vi "TrendsD03.vi"() -> ()   [LabVIEW 2019, in "D03.lvlib"]
uses:
  D03.lvlib
panel:
  out "No Change":bool
  out "Sudden Change":bool
  out "Decrease":bool
  out "Increase":bool
  out "Previous  ES":dbl
  out "Present  Speed":dbl
  out "Present Error":dbl format="%#.2g"
  out "Previous Error":dbl
  out "Previous  Speed":dbl
  out "Previous PW":dbl caption="Control Information"
  out "Pulse Trends":waveform(i16)[](graph) caption="Waveform Chart - Dark"
  in  "Close":bool
  out "disc name":string="Disc 03 Trends"
  out "dsgs":string="DSGS"
  out "Speed Trend":waveform(dbl)(graph) caption="Waveform Chart - Dark"
  out "Average Trend":waveform(dbl)[](graph) caption="Waveform Chart - Dark"
  out "Live Trend":waveform(dbl)[](graph) caption="Waveform Chart - Dark"
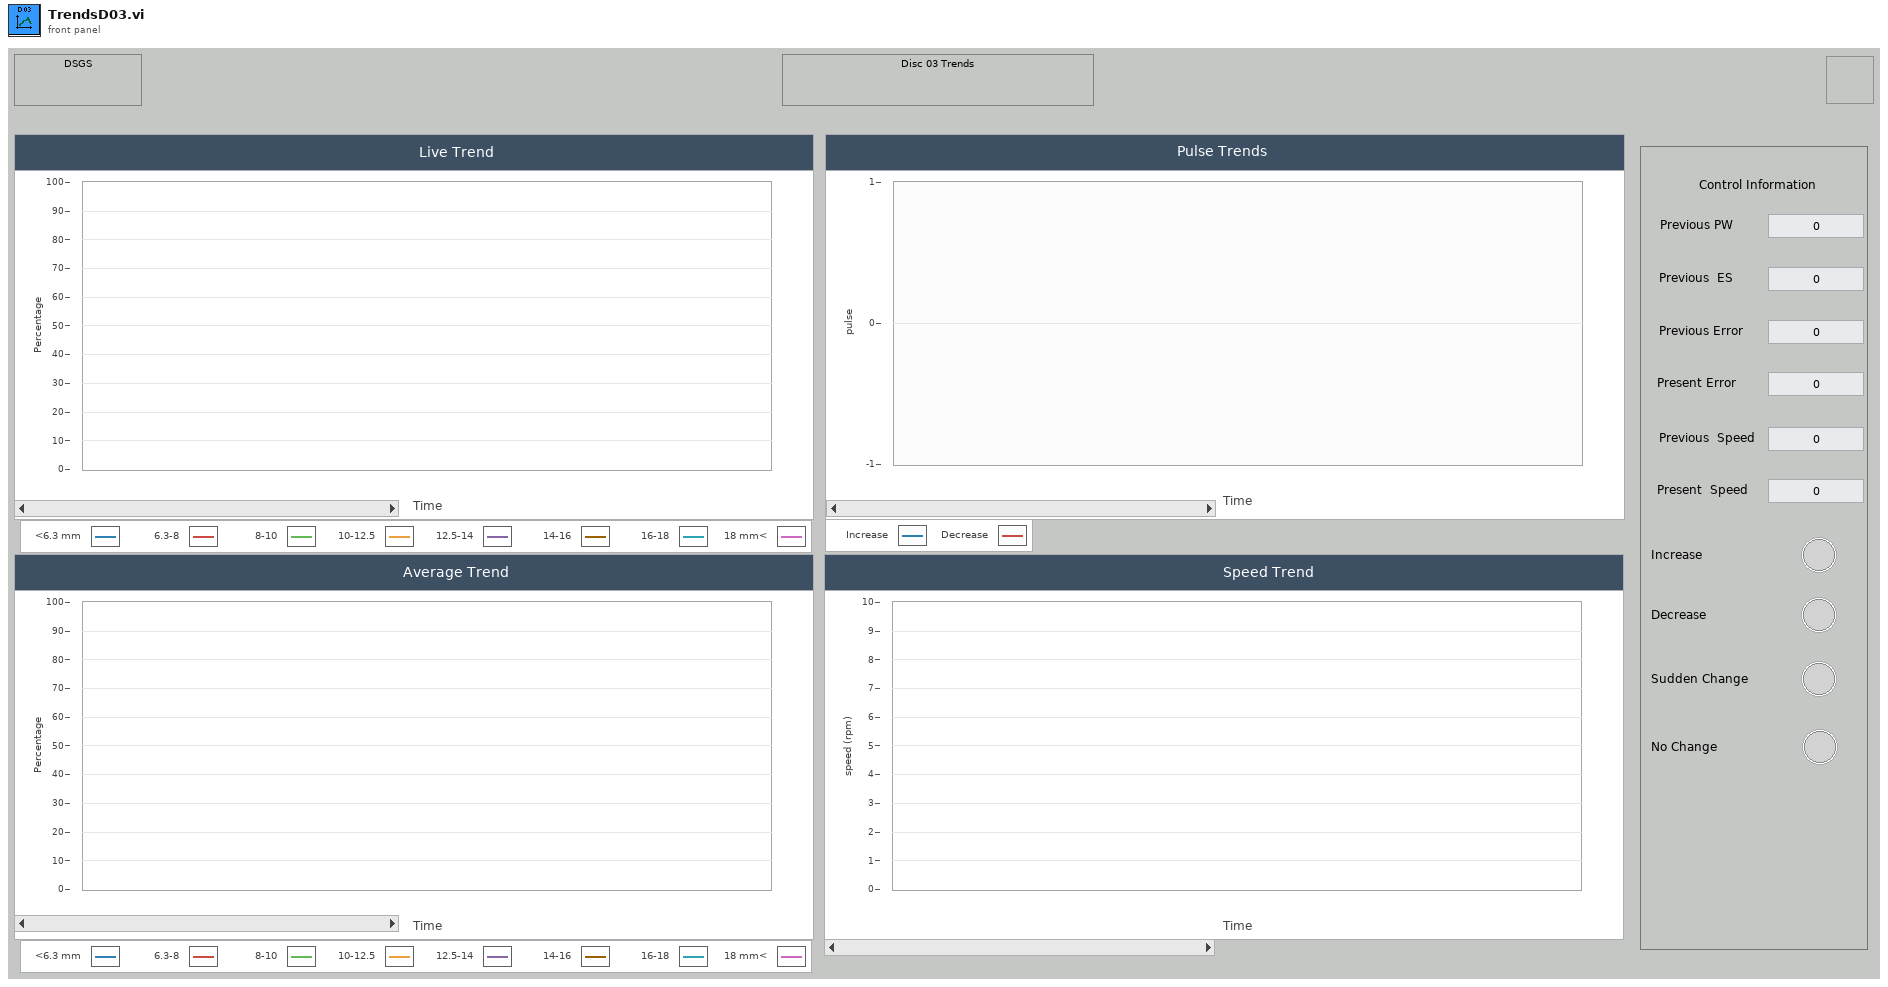
[diagram p1: front panel]
types:
  T1 = cluster{"decrease D28":bool, "increase D28":bool, "no change D28":bool, "sudden change D28":bool, "last error 28":dbl, "previous speed D28":dbl, "pulse width D28":dbl, "slope D28":dbl}
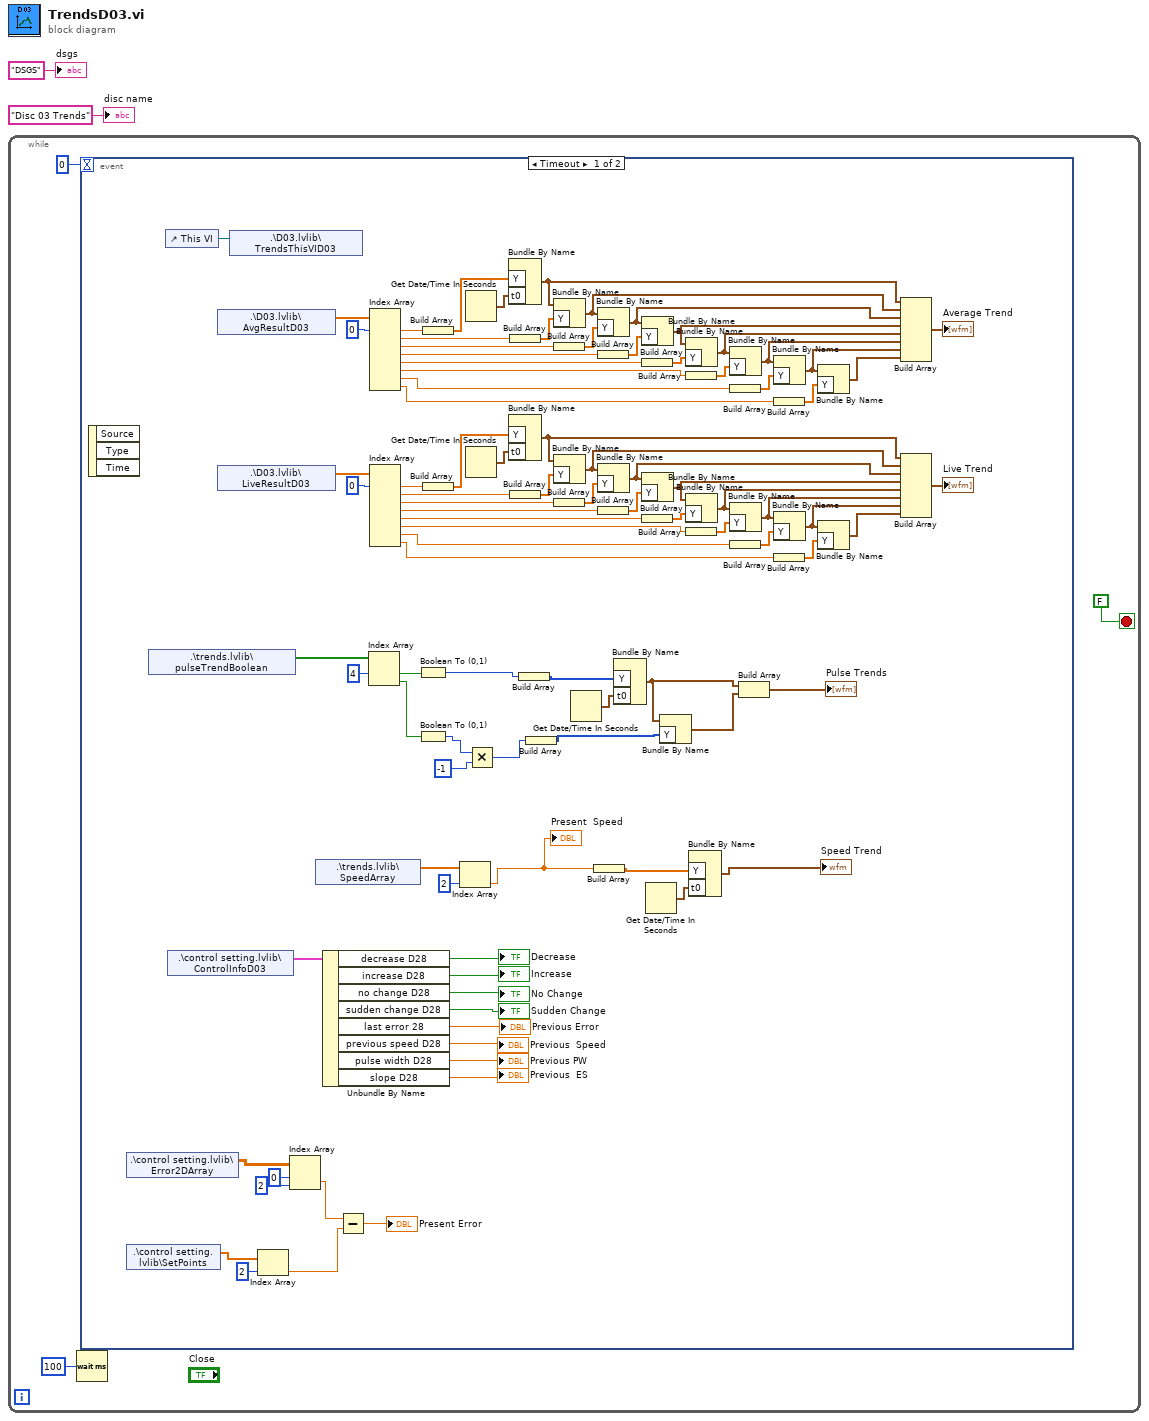
[diagram p0: block diagram]
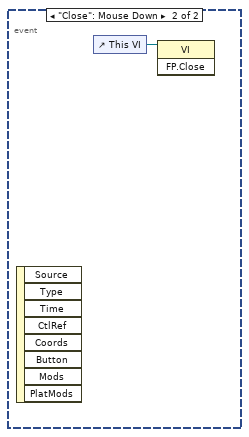
[diagram p2: hidden frame]
diagram:
  n1 = while {
    stop <- FALSE stop-if-true
    n2 = Wait (ms)(milliseconds to wait=u32 100) -> ()  [unwired: 1 out]
    n3 = event shown="[0] Timeout" {
      selector: _ -> [_ _]
      dyn-events: _ -> [_ _]
      timeout: 0 -> [_ _]
      event Timeout {
        n4 = event-data() -> ()  [unwired: 1 in, 3 out]
        n5 = shared-variable ".\\control setting.lvlib\\Error2DArray"() -> (w15:dbl[][])  [unwired: 1 in, 1 out]
        n6 = shared-variable ".\\control setting.lvlib\\SetPoints"() -> (w12:dbl[])  [unwired: 1 in, 1 out]
        n7 = shared-variable ".\\trends.lvlib\\pulseTrendBoolean"() -> (w30:bool[])  [unwired: 1 in, 1 out]
        n8 = control-ref of="This VI"() -> (w43:refnum<vi>)
        n9 = shared-variable ".\\control setting.lvlib\\ControlInfoD03"() -> (w23:T1)  [unwired: 1 in, 1 out]
        n10 = shared-variable ".\\D03.lvlib\\AvgResultD03"() -> (w54:dbl[])  [unwired: 1 in, 1 out]
        n11 = shared-variable ".\\D03.lvlib\\LiveResultD03"() -> (w99:dbl[])  [unwired: 1 in, 1 out]
        n12 = shared-variable ".\\D03.lvlib\\TrendsThisVID03"(w43) -> ()  [unwired: 1 in, 1 out]
        n13 = Index Array(array=w12, index=2) -> (element=w9:dbl)
        n14 = Index Array(array=w15, index (row)=0, index (col)=2 ("disabled index (col)")) -> (element=w10:dbl)
        n15 = shared-variable ".\\trends.lvlib\\SpeedArray"() -> (w28:dbl[])  [unwired: 1 in, 1 out]
        n16 = Unbundle By Name(w23) -> ("decrease D28"=→"Decrease":bool, "increase D28"=→"Increase":bool, "no change D28"=→"No Change":bool, "sudden change D28"=→"Sudden Change":bool, "last error 28"=→"Previous Error":dbl, "previous speed D28"=→"Previous  Speed":dbl, "pulse width D28"=→"Previous PW":dbl, "slope D28"=→"Previous  ES":dbl)
        n17 = Subtract(x=w10, y=w9) -> (x-y=→"Present Error":dbl)
        n18 = Index Array(array=w30, index #1=4 ("index")) -> (element #1=w31:bool, element #2=w38:bool)  [unwired: 1 in]
        n19 = Index Array(array=w54, index #1=0 ("index")) -> (element #1=w64:dbl, element #2=w65:dbl, element #3=w67:dbl, element #4=w69:dbl, element #5=w70:dbl, element #6=w72:dbl, element #7=w74:dbl, element #8=w53:dbl)  [unwired: 7 in]
        n20 = Index Array(array=w99, index #1=0 ("index")) -> (element #1=w89:dbl, element #2=w88:dbl, element #3=w86:dbl, element #4=w84:dbl, element #5=w83:dbl, element #6=w81:dbl, element #7=w79:dbl, element #8=w50:dbl)  [unwired: 7 in]
        n21 = Boolean To (0,1)(Boolean=w31) -> (0, 1=w39:i16)
        n22 = Boolean To (0,1)(Boolean=w38) -> (0, 1=w34:i16)
        n23 = Build Array(w64) -> (w75:dbl[])
        n24 = Build Array(w89) -> (w78:dbl[])
        n25 = Index Array(array=w28, index=2) -> (element=w6:dbl)
        "Present  Speed" <- w6
        n26 = Get Date/Time In Seconds() -> (seconds since 1Jan1904=w57:timestamp)
        n27 = Get Date/Time In Seconds() -> (seconds since 1Jan1904=w96:timestamp)
        n28 = Multiply(x=w34, y=i16 -1 ("0, 1")) -> (x*y=w32:i16)
        n29 = Bundle By Name("Y"=w75, "t0"=w57) -> (w63:waveform(dbl))  [unwired: 1 in]
        n30 = Bundle By Name("Y"=w78, "t0"=w96) -> (w90:waveform(dbl))  [unwired: 1 in]
        n31 = Build Array(w65) -> (w66:dbl[])
        n32 = Build Array(w88) -> (w87:dbl[])
        n33 = Build Array(w39) -> (w40:i16[])
        n34 = Build Array(w32) -> (w37:i16[])
        n35 = Bundle By Name(cluster=w63, "Y"=w66) -> (w62:waveform(dbl))
        n36 = Build Array(w67) -> (w68:dbl[])
        n37 = Bundle By Name(cluster=w90, "Y"=w87) -> (w91:waveform(dbl))
        n38 = Build Array(w86) -> (w85:dbl[])
        n39 = Get Date/Time In Seconds() -> (seconds since 1Jan1904=w41:timestamp)
        n40 = Build Array(w6) -> (w26:dbl[])
        n41 = Bundle By Name(cluster=w62, "Y"=w68) -> (w61:waveform(dbl))
        n42 = Build Array(w69) -> (w56:dbl[])
        n43 = Bundle By Name(cluster=w91, "Y"=w85) -> (w92:waveform(dbl))
        n44 = Build Array(w84) -> (w97:dbl[])
        n45 = Bundle By Name("Y"=w40, "t0"=w41) -> (w36:waveform(i16))  [unwired: 1 in]
        n46 = Bundle By Name(cluster=w61, "Y"=w56) -> (w60:waveform(dbl))
        n47 = Build Array(w70) -> (w71:dbl[])
        n48 = Bundle By Name(cluster=w92, "Y"=w97) -> (w93:waveform(dbl))
        n49 = Build Array(w83) -> (w82:dbl[])
        n50 = Get Date/Time In Seconds() -> (seconds since 1Jan1904=w25:timestamp)
        n51 = Bundle By Name(cluster=w36, "Y"=w37) -> (w35:waveform(i16))
        n52 = Bundle By Name(cluster=w60, "Y"=w71) -> (w59:waveform(dbl))
        n53 = Build Array(w72) -> (w73:dbl[])
        n54 = Bundle By Name(cluster=w93, "Y"=w82) -> (w94:waveform(dbl))
        n55 = Build Array(w81) -> (w80:dbl[])
        n56 = Bundle By Name("Y"=w26, "t0"=w25) -> (→"Speed Trend":waveform(dbl))  [unwired: 1 in]
        n57 = Bundle By Name(cluster=w59, "Y"=w73) -> (w58:waveform(dbl))
        n58 = Build Array(w74) -> (w76:dbl[])
        n59 = Bundle By Name(cluster=w94, "Y"=w80) -> (w95:waveform(dbl))
        n60 = Build Array(w79) -> (w77:dbl[])
        n61 = Build Array(w36, w35) -> (→"Pulse Trends":waveform(i16)[])
        n62 = Bundle By Name(cluster=w58, "Y"=w76) -> (w46:waveform(dbl))
        n63 = Build Array(w53) -> (w52:dbl[])
        n64 = Bundle By Name(cluster=w95, "Y"=w77) -> (w47:waveform(dbl))
        n65 = Build Array(w50) -> (w49:dbl[])
        n66 = Bundle By Name(cluster=w46, "Y"=w52) -> (w51:waveform(dbl))
        n67 = Bundle By Name(cluster=w47, "Y"=w49) -> (w48:waveform(dbl))
        n68 = Build Array(w63, w62, w61, w60, w59, w58, w46, w51) -> (→"Average Trend":waveform(dbl)[])
        n69 = Build Array(w90, w91, w92, w93, w94, w95, w47, w48) -> (→"Live Trend":waveform(dbl)[])
      }
      event "Close": Mouse Down {
        n70 = event-data() -> ()  [unwired: 1 in, 8 out]
        n71 = control-ref of="This VI"() -> (w100:refnum<vi>)
        n72 = invoke class="VI" method="FP.Close"(reference=w100) -> ()  [unwired: 2 in, 3 out]
      }
    }
  }
  "dsgs" <- "DSGS" ("dsgs")
  "disc name" <- "Disc 03 Trends" ("disc name")
